vi "CoolProp_SI_V2009.vi"(4 "Value2":dbl, 5 "Value1":dbl, 6 "Input Variable #2":T1(ring), 7 "Input Variable #1":T2(ring), 8 "error in (no error)":errorcluster, 9 "Output":string, 10 "Fluid":string, 11 "path in":path) -> (0 "error out":errorcluster, 2 "error_message":string, 3 "Return Value":dbl)   [LabVIEW 2009]
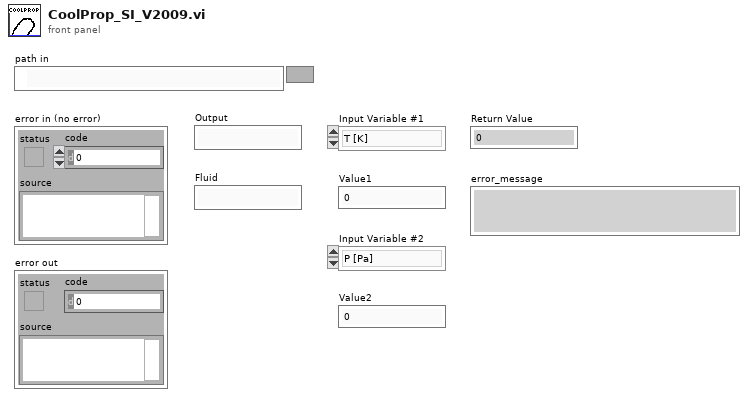
[diagram p1: front panel]
types:
  T1 = enum16{"P [Pa]", "D [kg/m3]", "Q [–]", "H [J/kg]", "S [J/kg-K]"}
  T2 = enum16{"T [K]", "P [Pa]", "H [J/kg]", "S [J/kg-K]"}
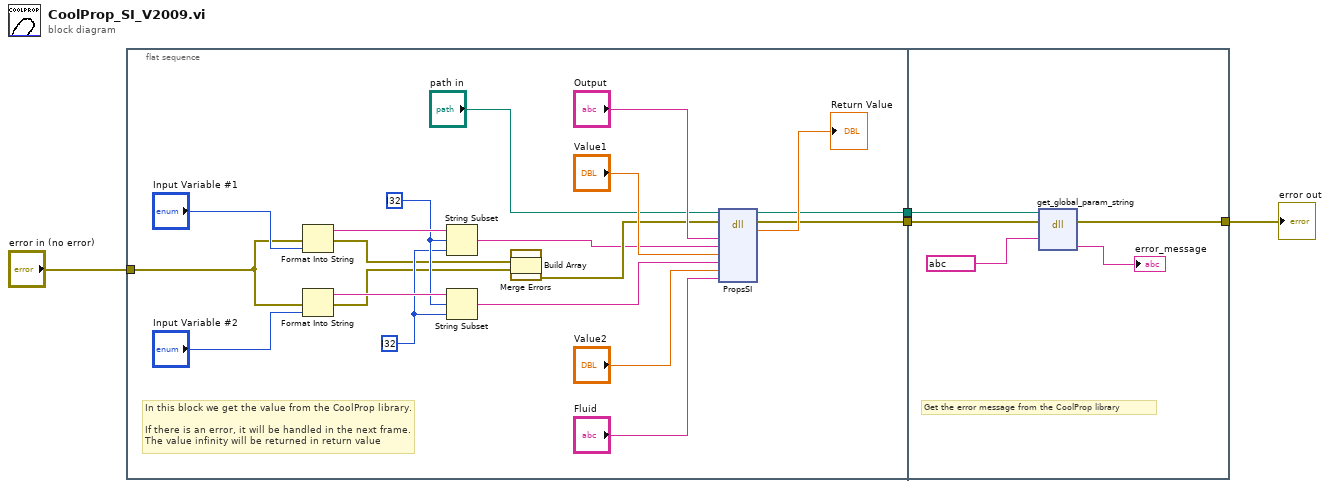
[diagram p0: block diagram]
diagram:
  n1 = flat-sequence {
    tunnel: "error in (no error)" -> [w9]
    tunnel: [w8] -> w3
    tunnel: [w7] -> w1
    tunnel: w3 -> [w28]
    tunnel: [w27] -> w2
    tunnel: w1 -> [w26]
    frame #0 {
      w17 = i32 ? ("length (rest)")
      w18 = i32 ? ("offset (0)")
      # "In this block we get the value from the CoolProp library.\n\nIf there is an error, it will be handled in the next frame.\nThe value infinity will be returned in return value"
      n2 = Format Into String(error in=w9, "Input Variable #1") -> (resulting string=w20:string, error out=w16:errorcluster)  [unwired: 2 in]
      n3 = Format Into String(error in=w9, "Input Variable #2") -> (resulting string=w19:string, error out=w15:errorcluster)  [unwired: 2 in]
      n4 = String Subset(string=w20, offset (0)=w18, length (rest)=w17) -> (substring=w11:string)
      n5 = String Subset(string=w19, offset (0)=w18, length (rest)=w17) -> (substring=w10:string)
      n6 = Build Array(w16, w15) -> (w5:errorcluster[])
      n7 = call <vilib>:"Merge Errors.vi"("error array in"=w5) -> ("error out"=w14:errorcluster)  [unwired: 6 in]
      n8 = dll-call lib="C:/Program Files (x86)/National Instruments/LabVIEW 2015/user.lib/CoolProp.dll" fn="PropsSI"(path in="path in", error in=w14, "Output"="Output", "Input1"=w11, "Value1"="Value1", "Input2"=w10, "Value2"="Value2", "Fluid"="Fluid") -> (path out=w7:path, error out=w8:errorcluster, "OutputValue"=→"Return Value":dbl)  [unwired: 7 in]
    }
    frame #1 {
      # "Get the error message from the CoolProp library"
      n9 = dll-call lib="C:/Program Files (x86)/National Instruments/LabVIEW 2011/user.lib/CoolProp.dll" fn="get_global_param_string"(path in=w26, error in=w28, "param"=string ?) -> (error out=w27:errorcluster, "error_message"=→"error_message":string)  [unwired: 2 in, 3 out]
    }
  }
  "error out" <- w2
